vi "Check Update Backlog.vi"(7 "TimingEngine":T1, 8 "error in (no error)":errorcluster, 11 "Cfg Grandmaster in":refnum<class "Cfg Grandmaster.lvclass">) -> (0 "error out":errorcluster, 3 "Cfg Grandmaster out":refnum<class "Cfg Grandmaster.lvclass">)   [LabVIEW 2018, in "Configuration Grandmaster.lvlib" / "Cfg Grandmaster.lvclass"]
uses:
  Cfg Grandmaster.lvclass
  Common/Controls/TE_Designator.ctl
  Cfg Grandmaster.lvclass/Cfg Grandmaster.ctl
  Class FP Ctrls/FP Controls.lvclass
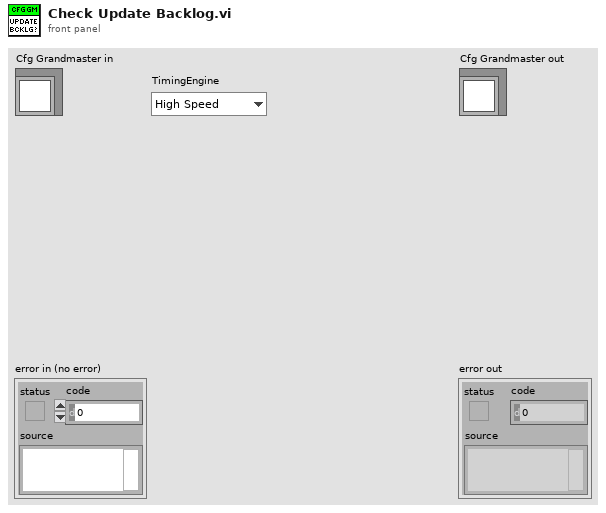
[diagram p1: front panel]
types:
  T1 = typedef "TE_Designator.ctl" = enum16{"High Speed", "Low Speed"}
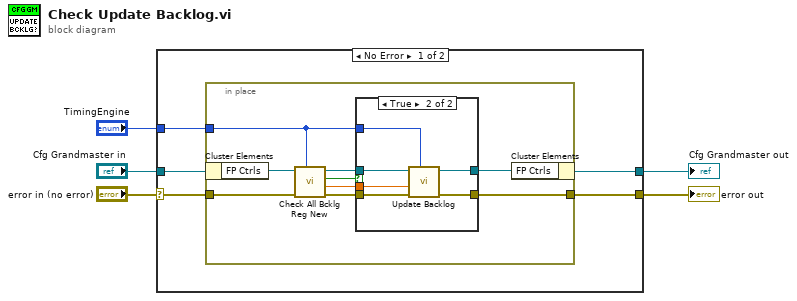
[diagram p0: block diagram]
diagram:
  n1 = case shown="No Error" "error in (no error)" {
    selector: "error in (no error)" -> [w10 w29]
    tunnel: [w6 w29] -> w4
    tunnel: [w7 w28] -> w2
    tunnel: "Cfg Grandmaster in" -> [w9 w28]
    tunnel: "TimingEngine" -> [w8 _]
    frame No Error {
      n2 = in-place {
        in-place-border: w10 -> [w19]
        in-place-border: w8 -> [w13]
        in-place-border: [w11] -> w6
        n3 = in-place-cluster #1(w9) -> ("FP Ctrls"=w14:refnum<class "FP Controls.lvclass">)
        n4 = call "Check All Bcklg Reg New.vi"("TimingEngine"=w13, "error in (no error)"=w19, "FP Controls in"=w14) -> ("error out"=w17:errorcluster, "Max Bcklg"=w16:dbl, "Update FP?"=w15:bool, "FP Controls out"=w18:refnum<class "FP Controls.lvclass">)  [unwired: 5 in]
        n5 = case shown="True" w15 {
          tunnel: w18 -> [w21 w27]
          tunnel: w17 -> [w20 w26]
          tunnel: w16 -> [_ w25]
          tunnel: [w21 w24] -> w12
          tunnel: [w20 w23] -> w11
          tunnel: w13 -> [_ w22]
          frame False {
          }
          frame True {
            n6 = call "Update Backlog.vi"("TimingEngine"=w22, "error in (no error)"=w26, "Backlog"=w25, "FP Controls in"=w27) -> ("error out"=w23:errorcluster, "FP Controls out"=w24:refnum<class "FP Controls.lvclass">)  [unwired: 6 in]
          }
        }
        n7 = in-place-cluster #1("FP Ctrls"=w12) -> (w7:refnum<class "Cfg Grandmaster.lvclass">)
      }
    }
    frame Error {
    }
  }
  "error out" <- w4
  "Cfg Grandmaster out" <- w2
